vi "Run Measurement.vi"(8 "error in (no error)":errorcluster, 11 "Operator UI in":refnum<class "Measurement UI.lvclass">) -> (0 "error out":errorcluster, 3 "Operator UI out":refnum<class "Measurement UI.lvclass">)   [LabVIEW 2015, in "Measurement UI.lvlib" / "Measurement UI.lvclass"]
uses:
  Measurement UI.lvclass
  <vilib>/ActorFramework/Actor/Actor.lvclass/Actor.ctl
  <vilib>/ActorFramework/Message Enqueuer/Message Enqueuer.lvclass/Message Enqueuer.ctl
  <vilib>/ActorFramework/Message Enqueuer/Init from Existing Queue.vi
  <vilib>/ActorFramework/Message Enqueuer/Message Enqueuer.lvclass
  Controller/Messages/Launch Measurements Message/Launch Measurements Message.lvclass
  User Interface/Messages/Update Status Display/Update Status Display.lvclass
  <vilib>/ActorFramework/Actor/Actor.lvclass
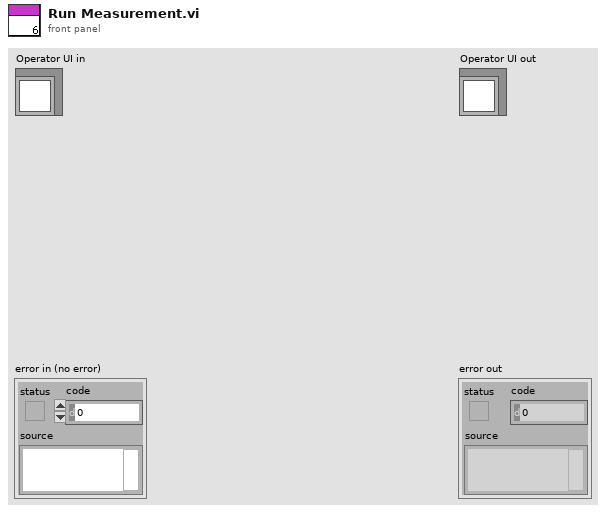
[diagram p1: front panel]
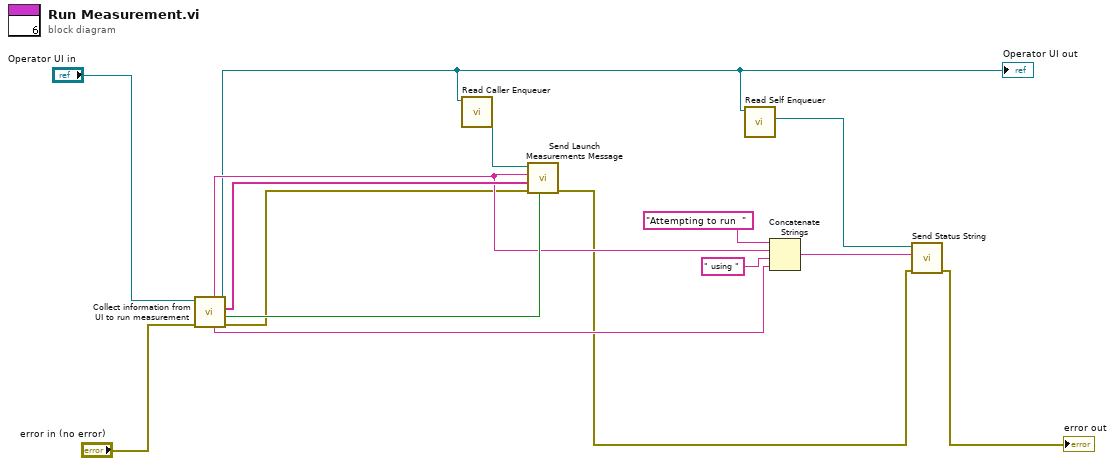
[diagram p0: block diagram]
diagram:
  n1 = call "Collect information from UI to run measurement.vi"("error in (no error)"="error in (no error)", "Measurement UI in"="Operator UI in") -> ("error out"=w2:errorcluster, "Show UI?"=w14:bool, "Device Names"=w15:string[], "Measurement UI out"=w4:refnum<class "Measurement UI.lvclass">, "String"=w9:string, "Measurement Name"=w12:string)  [unwired: 4 in]
  "Operator UI out" <- w4
  n2 = call <vilib>:"Read Caller Enqueuer.vi"("Actor"=w4) -> ("Caller Enqueuer"=w8:refnum<class "Message Enqueuer.lvclass">)  [unwired: 10 in]
  n3 = call "Send Launch Measurements Message.vi"("Show FP?"=w14, "error in (no error)"=w2, "Device Names"=w15, "Measurement Name"=w12, "Self Enqueuer In"=w8) -> ("error out"=w1:errorcluster)  [unwired: 5 in, 1 out]
  n4 = call <vilib>:"Read Self Enqueuer.vi"("Actor"=w4) -> ("Self Enqueuer"=w7:refnum<class "Message Enqueuer.lvclass">)  [unwired: 10 in]
  n5 = Concatenate Strings("Attempting to run  " ("string"), w12, " using " ("string"), w9) -> (w10:string)
  n6 = call "Send Status String.vi"("error in (no error)"=w1, "String"=w10, "Message Enqueuer in"=w7) -> ("error out"=→"error out":errorcluster)  [unwired: 7 in, 1 out]
